vi "HardwarePresent.vi"() -> ()   [LabVIEW 2012]
panel:
  in  "HardwarePresent":bool
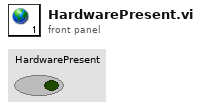
[diagram p1: front panel]
diagram:
